vi "simple VISA.vi"() -> ()   [LabVIEW 2017]
panel:
  in  "VISA resource name":refnum<visa-resource-name>
  in  "write buffer":string
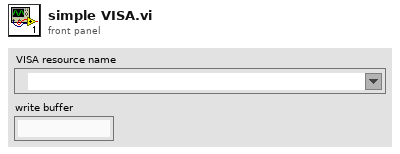
[diagram p1: front panel]
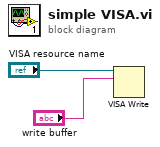
[diagram p0: block diagram]
diagram:
  n1 = VISA Write(VISA resource name="VISA resource name", write buffer="write buffer") -> ()  [unwired: 1 in, 3 out]
